vi "Anritsu VNA Read Frequency On-Off.vi"(7 "Anritsu VNA":T1, 8 "error in (no error)":errorcluster, 11 "VISA Resource Name":refnum<visa-resource-name>) -> (0 "error out":errorcluster, 2 "Frequencies Blanked":bool, 3 "dup VISA Resource Name":refnum<visa-resource-name>)   [LabVIEW 2011]
doc: "This VI for the HP8753B Network Analyzers reads the stimulus values. Except when performing log sweeps and freq list sweeps, this VI uses the start and stop values and the number of points to calcuate the stimulus values."
uses:
  TypeDefs/Anritsu VNA Instrument Info.ctl
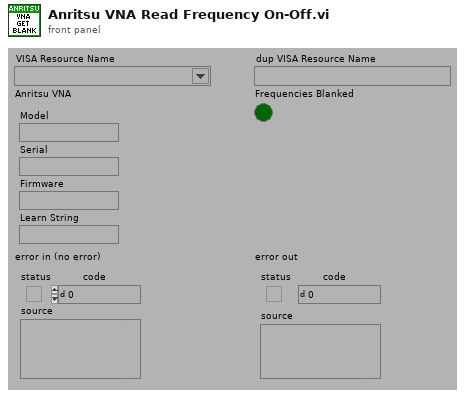
[diagram p1: front panel]
types:
  T1 = typedef "Anritsu VNA Instrument Info.ctl" = cluster{"Model":string, "Serial":string, "Firmware":string, "Learn String":string}
  T2 = typedef "Anritsu VNA Model.ctl" = enum16{"Not Supported", "37XXXX", "MS20XXX", "MS462XX", "MS464XX"}
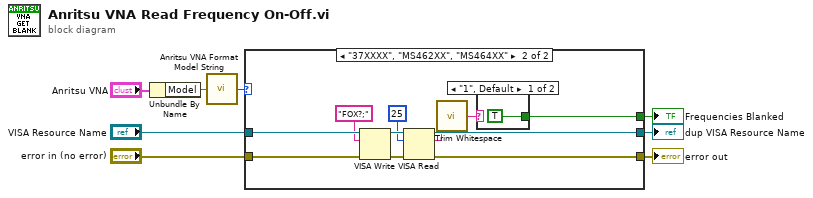
[diagram p0: block diagram]
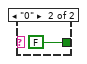
[diagram p3: hidden frame]
diagram:
  n1 = Unbundle By Name("Anritsu VNA") -> ("Model"=w2:string)
  n2 = call "Anritsu VNA Format Model String.vi"("Model"=w2) -> ("Model"=w1:T2)
  n3 = case shown="\"37XXXX\", \"MS462XX\", \"MS464XX\"" w1 {
    tunnel: [w10 w17] -> w8
    tunnel: [w9 w16] -> w7
    tunnel: "error in (no error)" -> [w9 w19]
    tunnel: "VISA Resource Name" -> [w10 w18]
    tunnel: [_ w11] -> w3
    frame "Not Supported", "MS20XXX" {
      # "These VNAs do not have the ability to blank the frequencies."
    }
    frame "37XXXX", "MS462XX", "MS464XX" {
      n4 = VISA Write(VISA resource name=w18, write buffer="FOX?;", error in (no error)=w19) -> (VISA resource name out=w20:refnum<visa-resource-name>, error out=w21:errorcluster)  [unwired: 1 out]
      n5 = VISA Read(VISA resource name=w20, byte count=u32 25, error in (no error)=w21) -> (VISA resource name out=w17:refnum<visa-resource-name>, read buffer=w13:string, error out=w16:errorcluster)  [unwired: 1 out]
      n6 = call <vilib>:"Trim Whitespace.vi"("string"=w13) -> ("trimmed string"=w12:string)  [unwired: 1 in]
      n7 = case shown="\"1\", Default" w12 {
        tunnel: [TRUE ("Blank Frequencies") FALSE ("Blank Frequencies")] -> w11
        frame "1", Default {
        }
        frame "0" {
        }
      }
    }
  }
  "dup VISA Resource Name" <- w8
  "error out" <- w7
  "Frequencies Blanked" <- w3
